vi "Extract Numbers with Match Pattern.vi"(11 "String":string="one 2 -3 4.0 5.5") -> (3 "Numeric":dbl)   [LabVIEW 2022 SP3]
doc: "Uses the Match Pattern function to find all numbers in the given string, and returns them in an array. All of the following formats are recognized:\n\n123 1.23 .123 0.123 -1.23\n\nNo spaces or other characters may appear within the number, but any characters may appear before or after the number. This example assumes that the input string contains periods and not commas for the decimal separator."
panel:
  # "Overview: Demonstrates how to use the Match Pattern function to extract numeric values from a string.\nInstructions:\n1. Specify a String value containing numbers.\n2. Run the VI. All numbers in the String are displayed in the Extracted Numbers array."
  # "Note: Numbers that are spelled out (like \"one\" in the string above) are not interpreted as numbers.  Scientific notation is also not handled by this example. Additionally, this example will only extract decimal numbers from the string that use the \".\" character as a decimal separator."
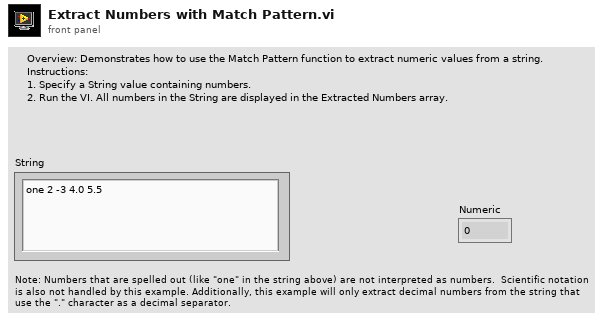
[diagram p1: front panel]
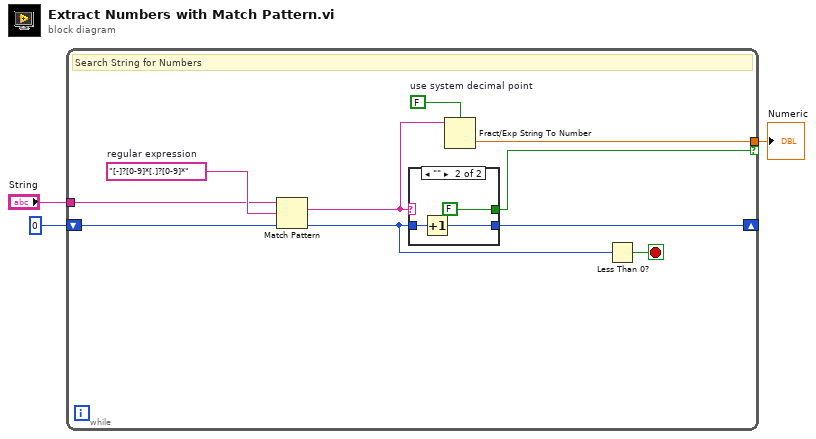
[diagram p0: block diagram]
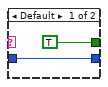
[diagram p2: hidden frame]
diagram:
  n1 = while {
    shift-left: 0 -> [w9]
    shift-right: [w4] -> _
    tunnel: [w13] -> w1 if=w6
    tunnel: "String" -> [w8]
    stop <- w12 stop-if-true
    w11 = FALSE  # use system decimal point
    w10 = "[-]?[0-9]*[.]?[0-9]*"  # regular expression
    # "Search String for Numbers"
    n2 = Match Pattern(string=w8, regular expression=w10, offset (0)=w9) -> (match substring=w7:string, offset past match=w5:i32)  [unwired: 2 out]
    n3 = case shown="\"\"" w7 {
      tunnel: [w15 w17] -> w4
      tunnel: [TRUE FALSE] -> w6
      tunnel: w5 -> [w15 w18]
      frame Default {
      }
      frame "" {
        n4 = Increment(x=w18) -> (x+1=w17:i32)
      }
    }
    n5 = Fract/Exp String To Number(use system decimal point (T)=w11, string=w7) -> (number=w13:dbl)  [unwired: 2 in, 1 out]
    n6 = Less Than 0?(x=w5) -> (x < 0?=w12:bool)
  }
  "Numeric" <- w1
